vi "GlobalDrivebase.vi"() -> ()   [LabVIEW 2020]
panel:
  out "SEN_Drive_Fault":bool[](array[boolean])
  out "DAT_Unlock_Azimuth":bool
  out "OUT_Azimuth_Error_3 (deg)":dbl
  out "OUT_Azimuth_Error_1 (deg)":dbl
  out "OUT_Azimuth_Error_2 (deg)":dbl
  out "OUT_Azimuth_Error_0 (deg)":dbl
  out "SEN_Drive_Raw_Velocity_2 (rpm)":dbl
  out "SEN_Drive_Raw_Velocity_3 (rpm)":dbl
  out "SEN_Drive_Raw_Velocity_1 (rpm)":dbl
  out "SEN_Drive_Raw_Velocity_0 (rpm)":dbl
  out "DAT_Hopper_Sensor_Override":bool
  out "DAT_Auto_Targeting_Override":bool
  out "SEN_Azimuth_Position_Unwrapped_3 (deg)":dbl
  out "SEN_Azimuth_Position_Unwrapped_2 (deg)":dbl
  out "SEN_Azimuth_Position_Unwrapped_1 (deg)":dbl
  out "SEN_Azimuth_Position_Unwrapped_0 (deg)":dbl
  out "SEN_Latched_Shift_Time_3 (ms)":u32
  out "SEN_Latched_Shift_Time_2 (ms)":u32
  out "SEN_Latched_Shift_Time_1 (ms)":u32
  out "SEN_Latched_Shift_Time_0 (ms)":u32
  out "SEN_Shifter_Stuck":bool[](array[boolean])
  out "SEN_Shifter_Failure":bool[](array[boolean])
  in  "SEN_Actual_Shifter_State_3":T1(ring)
  in  "SEN_Actual_Shifter_State_2":T1(ring)
  in  "SEN_Actual_Shifter_State_1":T1(ring)
  in  "SEN_Actual_Shifter_State_0":T1(ring)
  out "SEN_Drive_Velocity_2 (ft/s)":dbl
  out "SEN_Drive_Velocity_3 (ft/s)":dbl
  out "SEN_Drive_Velocity_1 (ft/s)":dbl
  out "SEN_Drive_Velocity_0 (ft/s)":dbl
  out "SEN_Drive_Overheat":bool[](array[boolean])
  out "SEN_Azimuth_Fault":bool[](array[boolean])
  out "SEN_Drive_Temp_2 (C)":u8
  out "SEN_Drive_Temp_3 (C)":u8
  out "SEN_Drive_Temp_1 (C)":u8
  out "SEN_Drive_Temp_0 (C)":u8
  out "SEN_Azimuth_Position_3 (deg)":dbl
  out "SEN_Azimuth_Position_2 (deg)":dbl
  out "SEN_Azimuth_Position_1 (deg)":dbl
  out "SEN_Azimuth_Position_0 (deg)":dbl
  out "OUT_Orientation Mode":enum16{"Robot-Oriented", "Field-Oriented"}(ring)
  out "OUT_Current_Driver_Profile_Setpoints":dbl[](array[numeric])
  out "OUT_Force_Low_Gear":bool
  out "OUT_High_Gear_Requested_2":bool
  out "OUT_High_Gear_Requested_1":bool
  out "OUT_High_Gear_Requested_3":bool
  out "OUT_High_Gear_Requested_0":bool
  out "OUT_Azimuth_Goal_3 (deg)":dbl
  out "OUT_Azimuth_Goal_1 (deg)":dbl
  out "OUT_Azimuth_Goal_2 (deg)":dbl
  out "OUT_Azimuth_Goal_0 (deg)":dbl
  out "OUT_Swerve_Rotation_Command":dbl
  out "OUT_Drive_Mode":enum16{"Driver Control", "Lock Heading"}(ring)
  out "OUT_Boost_Drive_Train":bool
  out "OUT_Drive_Command_3":dbl
  out "OUT_Drive_Command_1":dbl
  out "OUT_Drive_Command_2":dbl
  out "OUT_Drive_Command_0":dbl
  out "CON_Legal_Drivers":string[](array[string])
  out "DAT_New_Driver_Profile_Setpoints":dbl[](array[numeric])
  out "DAT_Apply_Driver_Profile_Setpoints":bool
  out "DAT_Starting_IMU_Reset":bool
  out "DAT_Field_Oriented_Override":bool
  out "DAT_Home_Wheels":bool
  out "DAT_Calibrate_Wheels":bool
  out "CON_Max_Robot_Rotation_Speed_(deg/s)":dbl
  out "CON_Max_Robot_Low_Gear_Speed_(ft/s)":dbl
  out "CON_Azimuth_Gear_Ratio":dbl
  out "CON_Drive_High_Gear_Ratio":dbl
  out "CON_Drive_Low_Gear_Ratio":dbl
  out "CON_Drive_Wheel_Diameter (in)":dbl
  out "CON_Robot_Width_Bumpers (in)":dbl
  out "CON_Robot_Length_Bumpers (in)":dbl
  out "CON_Robot_Minimum_Dimension (in)":dbl
  out "CON_Robot_Width (in)":dbl
  out "CON_Robot_Length (in)":dbl
  out "CON_Max_Robot_Ground_Speed_(ft/s)":dbl
  out "REF_Shifter_2":string
  out "REF_Shifter_1":string
  out "REF_Shifter_0":string
  out "REF_Shifter_3":string
  out "REF_Azimuth_3":string
  out "REF_Azimuth_2":string
  out "REF_IMU_0":string
  out "REF_Azimuth_1":string
  out "REF_Azimuth_0":string
  out "REF_Drive_3":string
  out "REF_Drive_2":string
  out "REF_Drive_1":string
  out "REF_Drive_0":string
  # "SENSORS"
  # "OUTPUTS"
  # "DRIVER STATION DATA"
  # "DEVICE REFERENCE NAMES"
  # "CONSTANTS"
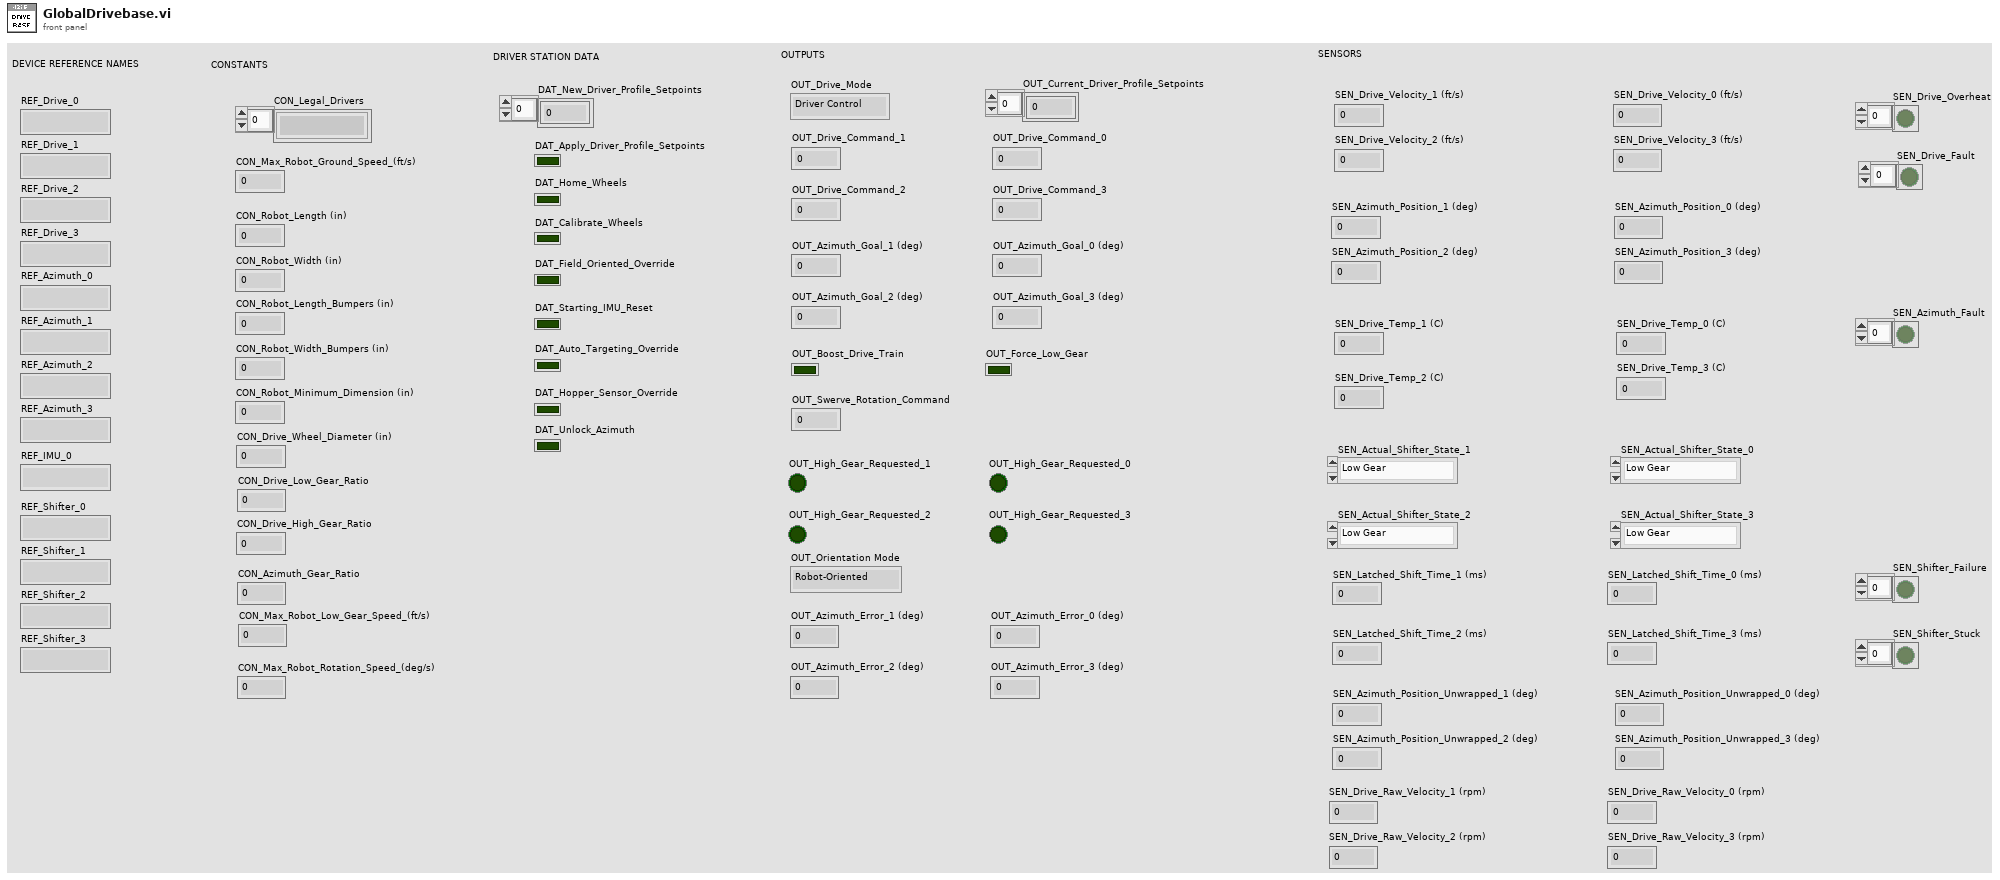
[diagram p1: front panel]
types:
  T1 = enum16{"Low Gear", "High Gear", "Transiting", "Unknown", "Force Low Gear"}
diagram:
